vi "Supply_SetVolts.vi"(8 "error in (no error)":errorcluster, 9 "Command string":string, 10 "Volts IN [V]":dbl, 11 "KE236 in":refnum<class "KE236.lvclass">) -> (0 "error out":errorcluster, 2 "Compliance exceeded?":bool, 3 "KE236 out":refnum<class "KE236.lvclass">)   [LabVIEW 2018, in "KE236.lvclass"]
uses:
  KE236.lvclass
  SupplyControl.lvclass
panel:
  out "Command sent":string
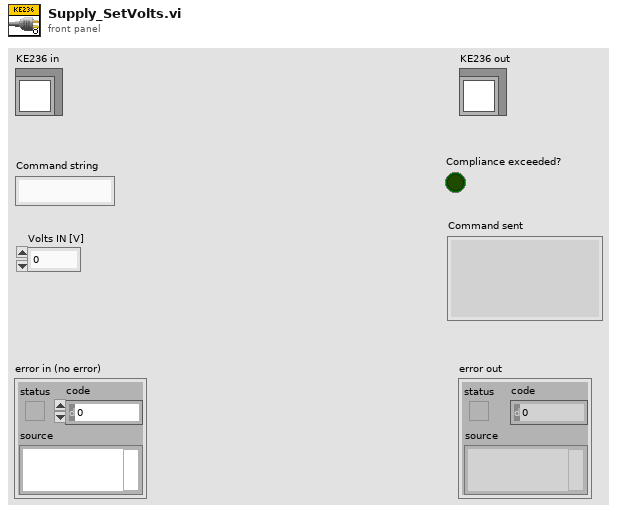
[diagram p1: front panel]
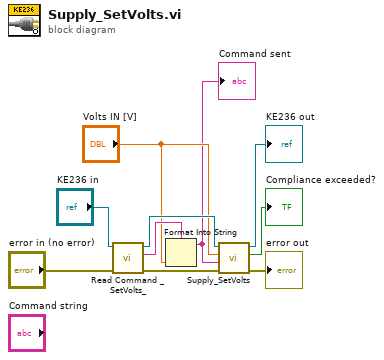
[diagram p0: block diagram]
diagram:
  n1 = call-dynamic "Read Command _SetVolts_.vi"("error in (no error)"="error in (no error)", "SupplyControl in"="KE236 in") -> ("error out"=w4:errorcluster, "Command \"SetVolts\""=w5:string, "SupplyControl out"=w3:refnum<class "KE236.lvclass">)  [unwired: 7 in]
  n2 = Format Into String(format string=w5, "Volts IN [V]") -> (resulting string=w1:string)  [unwired: 2 in, 1 out]
  "Command sent" <- w1
  n3 = call-parent "Supply_SetVolts.vi"("error in (no error)"=w4, "Command string"=w1, "Volts IN [V]"="Volts IN [V]", "SupplyControl in"=w3) -> ("error out"=→"error out":errorcluster, "Compliance exceeded?"=→"Compliance exceeded?":bool, "SupplyControl out"=→"KE236 out":refnum<class "KE236.lvclass">)  [unwired: 5 in]
